vi "Sequence Dialog.vi"(8 "error in (no error)":errorcluster, 10 "Sequence UI":refnum<queue>, 11 "State Cluster In":T3 {"Main Config"."PR Module Configs"."Settings"."PID 2 Parameters"."output range"."output low" format="%.2f"; "Main Config"."PR Module Configs"."Settings"."PID 2 Parameters"."output range"."output high" min=0.0 max=100.0 format="%.2f"; "Main Config"."PR Module Configs"."Settings"."PID 2 Parameters"."PID gains"."derivative time (Td, min)" format="%.3f"; "Main Config"."PR Module Configs"."Settings"."PID 2 Parameters"."PID gains"."integral time (Ti, min)" format="%.3f"; "Main Config"."PR Module Configs"."Settings"."PID 2 Parameters"."PID gains"."proportional gain (Kc)" format="%.3f"; "Main Config"."Steps"."Control" items=["Pump %", "Setpoint"]; "Main Config"."TCU Module Configs"."Settings"."Huber Unistat 410 Settings"."Address" min=0 max=99 format="%02.0f"; "Main Config"."TCU Module Configs"."Settings"."Julabo FP-50 Settings"."Pump Power" min=0 max=8 step=1; "Main Config"."TCU Module Configs"."Settings"."Lauda Settings"."Pump Power" min=0 max=8 step=1; "Main Config"."Flow Module Configs"."Settings"."Bronkhorst M14 Settings"."Smoothing Steps" min=1 step=1; "Main Config"."Flow Module Configs"."Settings"."Bronkhorst M13 Settings"."Smoothing Steps" min=1 step=1; "Main Config"."Pump Module Configs"."Settings"."Ismatech 3 Channel Settings"."Channel Number" min=0 max=3; "Main Config"."Pump Module Configs"."Settings"."Ismatech 3 Channel Settings"."Pump Number" min=1; "Main Config"."Pump Module Configs"."Settings"."ASIA Pump C"."channel" min=0 max=1 step=1; "Main Config"."Pump Module Configs"."Settings"."Masterflex"."Pump Number" min=1.0 max=20.0 step=1.0; "Main Config"."Pump Module Configs"."Settings"."Ismatech"."Pump Number" min=1.0 max=20.0 step=1.0; "Main Config"."Feed Module Configs"."Settings"."Bronkhorst M14 Settings"."Smoothing Steps" min=1 step=1; "Main Config"."Feed Module Configs"."Settings"."Ismatech 3 Channel Settings"."Channel Number" min=0 max=3; "Main Config"."Feed Module Configs"."Settings"."Ismatech 3 Channel Settings"."Pump Number" min=1; "Main Config"."Feed Module Configs"."Settings"."PID range"."PID Low" min=0.0 max=100.0 format="%.2f"; "Main Config"."Feed Module Configs"."Settings"."PID range"."PID High" format="%.2f"; "Main Config"."Feed Module Configs"."Settings"."PID 2 Parameters"."PID gains"."derivative time (Td, min)" format="%.3f"; "Main Config"."Feed Module Configs"."Settings"."PID 2 Parameters"."PID gains"."integral time (Ti, min)" format="%.3f"; "Main Config"."Feed Module Configs"."Settings"."PID 2 Parameters"."PID gains"."proportional gain (Kc)" format="%.3f"; "Main Config"."Feed Module Configs"."Settings"."Bronkhorst M13 Flow Meter"."Smoothing Steps" min=1 step=1; "Main Config"."Feed Module Configs"."Settings"."ASIA Pump C"."channel" min=0 max=1 step=1; "Main Config"."Feed Module Configs"."Settings"."Ismatech"."Pump Number" min=1.0 max=20.0 step=1.0; "Main Config"."Feed Module Configs"."Settings"."Masterflex"."Pump Number" min=1.0 max=20.0 step=1.0}) -> (0 "error out":errorcluster, 1 "Start":bool, 2 "cancelled":bool, 3 "State Cluster Out":T3 {"Main Config"."PR Module Configs"."Settings"."PID 2 Parameters"."output range"."output low" format="%.2f"; "Main Config"."PR Module Configs"."Settings"."PID 2 Parameters"."output range"."output high" min=0.0 max=100.0 format="%.2f"; "Main Config"."PR Module Configs"."Settings"."PID 2 Parameters"."PID gains"."derivative time (Td, min)" format="%.3f"; "Main Config"."PR Module Configs"."Settings"."PID 2 Parameters"."PID gains"."integral time (Ti, min)" format="%.3f"; "Main Config"."PR Module Configs"."Settings"."PID 2 Parameters"."PID gains"."proportional gain (Kc)" format="%.3f"; "Main Config"."Steps"."Control" items=["Pump %", "Setpoint"]; "Main Config"."TCU Module Configs"."Settings"."Huber Unistat 410 Settings"."Address" min=0 max=99 format="%02.0f"; "Main Config"."TCU Module Configs"."Settings"."Julabo FP-50 Settings"."Pump Power" min=0 max=8 step=1; "Main Config"."TCU Module Configs"."Settings"."Lauda Settings"."Pump Power" min=0 max=8 step=1; "Main Config"."Flow Module Configs"."Settings"."Bronkhorst M14 Settings"."Smoothing Steps" min=1 step=1; "Main Config"."Flow Module Configs"."Settings"."Bronkhorst M13 Settings"."Smoothing Steps" min=1 step=1; "Main Config"."Pump Module Configs"."Settings"."Ismatech 3 Channel Settings"."Channel Number" min=0 max=3; "Main Config"."Pump Module Configs"."Settings"."Ismatech 3 Channel Settings"."Pump Number" min=1; "Main Config"."Pump Module Configs"."Settings"."ASIA Pump C"."channel" min=0 max=1 step=1; "Main Config"."Pump Module Configs"."Settings"."Masterflex"."Pump Number" min=1.0 max=20.0 step=1.0; "Main Config"."Pump Module Configs"."Settings"."Ismatech"."Pump Number" min=1.0 max=20.0 step=1.0; "Main Config"."Feed Module Configs"."Settings"."Bronkhorst M14 Settings"."Smoothing Steps" min=1 step=1; "Main Config"."Feed Module Configs"."Settings"."Ismatech 3 Channel Settings"."Channel Number" min=0 max=3; "Main Config"."Feed Module Configs"."Settings"."Ismatech 3 Channel Settings"."Pump Number" min=1; "Main Config"."Feed Module Configs"."Settings"."PID range"."PID Low" min=0.0 max=100.0 format="%.2f"; "Main Config"."Feed Module Configs"."Settings"."PID range"."PID High" format="%.2f"; "Main Config"."Feed Module Configs"."Settings"."PID 2 Parameters"."PID gains"."derivative time (Td, min)" format="%.3f"; "Main Config"."Feed Module Configs"."Settings"."PID 2 Parameters"."PID gains"."integral time (Ti, min)" format="%.3f"; "Main Config"."Feed Module Configs"."Settings"."PID 2 Parameters"."PID gains"."proportional gain (Kc)" format="%.3f"; "Main Config"."Feed Module Configs"."Settings"."Bronkhorst M13 Flow Meter"."Smoothing Steps" min=1 step=1; "Main Config"."Feed Module Configs"."Settings"."ASIA Pump C"."channel" min=0 max=1 step=1; "Main Config"."Feed Module Configs"."Settings"."Ismatech"."Pump Number" min=1.0 max=20.0 step=1.0; "Main Config"."Feed Module Configs"."Settings"."Masterflex"."Pump Number" min=1.0 max=20.0 step=1.0}, 4 "Pause":bool, 5 "Abort":bool)   [LabVIEW 2018, in "Sequencing Library.lvlib"]
uses:
  Sequencing Library.lvlib
  Squence Control.ctl
  controls/Step Cluster.ctl
  Drag and Drop/State Cluster.ctl
  support/Message Queue/Message Cluster.ctl
  Drag and Drop/Thumbnail Cluster.ctl
  Drag and Drop/Object Cluster.ctl
  <vilib>/Utility/miscctls.llb/LVRectTypeDef.ctl
  Drag and Drop/Object Type Enum.ctl
  <vilib>/Utility/miscctls.llb/LVPositionTypeDef.ctl
  Config Module/Controls/Main Config Cluster.ctl
  OPC/OPC Module Config.ctl
  Scale Module Folder/Measure Instrument/State Enum.ctl
  <vilib>/Utility/miscctls.llb/LVPoint32TypeDef.ctl
  OPC/OPC Settings.ctl
  OPC/Variable Data Cluster.ctl
  <vilib>/OPCUA/controls/NodeId.ctl
  <vilib>/OPCUA/controls/OPC UA StatusCode.ctl
  <vilib>/OPCUA/controls/Subscription ID.ctl
  <vilib>/OPCUA/controls/OPC UA Client Refnum.ctl
  <vilib>/OPCUA/controls/Subscription Data Change.ctl
  <vilib>/OPCUA/controls/Data Type.ctl
  OPC/OPC Tag Data.ctl
  Feed Module/Controls/Feed Module Config Cluster.ctl
  Feed Module/Controls/Feed Module Settings Cluster.ctl
  Ismatec ISM 831C/Controls/Ismatech ISM831C Settings Cluster.ctl
  Masterflex 7550-30/Controls/Settings Cluster.ctl
  Mettler Toledo/Controls/Settings Cluster.ctl
  Bronkhorst M13 Flow Meter/Settings Cluster.ctl
  Measure Instrument/PID 2 Parameters Cluster.ctl
  Measure Instrument/PID Input Enum.ctl
  Measure Instrument/PID 2 Output Enum.ctl
  Tacmina QI/Tacmina QI DAQ Setting.ctl
  KNF Pump/Settings Cluster plus SIMDOS.ctl
  ASIA Pump/Pump Settings.ctl
  VICI M50 Party Mode/Settings Cluster.ctl
  FLOM Pump/Settings Cluster.ctl
  SSI PR Class/SSI PR or LD Settings Cluster.ctl
  Masterflex 75211/Masterflex 75211 DAQ Setting.ctl
  SSI PR Class/SSI P40 Settings Cluster.ctl
  Ismatec 78001/Ismatec 4083.ctl
  Bronkhorst M14 Flow Meter/Settings Cluster.ctl
  Tag VIs/Numeric Alarm Settings Cluster.ctl
  TT Module/Controls/TT Module Config Cluster.ctl
  Acquisition/Hardware Configuration.ctl
  Acquisition/Task Cluster.ctl
  PT Module/Controls/PT Module Config Cluster.ctl
  Scale Module Folder/Feed Module/Controls/Scale Module Config Cluster.ctl
  Scale Module Folder/Feed Module/Controls/Scale Module Settings Cluster.ctl
  Pump Module Folder/Pump Module Config Cluster.ctl
  Pump Module Folder/Pump Module Settings Cluster.ctl
  LabJack Module/Controls/U3 Module Config Cluster.ctl
  Decoration Module/Decoration Module Config Cluster.ctl
  Flow Module Folder/Feed Module/Controls/Flow Module Config Cluster.ctl
  Flow Module Folder/Feed Module/Controls/Flow Module Settings Cluster.ctl
  TCU Module/TCU Module Folder/TCU Module Config Cluster.ctl
  TCU Module/TCU Module Folder/TCU Module Settings Cluster.ctl
  TCU Module/TCU Module Folder/Measure Instrument/Output Devices.ctl
  Huber TCU/Huber Settings.ctl
  Lauda Integral XT-150 TCU/Lauda Settings.ctl
  Julabo Type 1 TCU/Julabo Type 1 TCU Folder/Julabo FP-50 Settings.ctl
  Huber Unistat 410 TCU/Huber Unistat 410 RS485 Settings.ctl
  D-O Module Folder/Not Sure Where this is Used.ctl
  D-O Module Folder/D-O Module Config Cluster.ctl
  D-O Module Folder/Valve Clusters.ctl
  D-O Module Folder/D-O Module Settings Cluster.ctl
  D-O Module Folder/D-O Device Settings Cluster.ctl
  VICI Electronic Actuator/VICI Electronic Actuator Settings.ctl
  Pressure Regulator Control Module/Pressure Regulator/Controls/4-20mA Module Config Cluster.ctl
  Pressure Regulator Control Module/Pressure Regulator/Controls/4-20mA Module Settings Cluster.ctl
  Pressure Transmitter/Pressure Transmitter Device Settings.ctl
  Pressure Reg Module/Pressure Regulator Device Settings.ctl
  Sonicator Module Folder/Feed Module/Controls/Sonicator Module Config Cluster.ctl
  Sonicator Module Folder/Feed Module/Controls/Sonicator Module Settings Cluster.ctl
  Sonic Systems P100/Sonic Systems P100 Settings.ctl
  Agitator Module Folder/Feed Module/Controls/Agitator Module Config Cluster.ctl
  Agitator Module Folder/Feed Module/Controls/Agitator Module Settings Cluster.ctl
  IKA EUROSTAR/IKA EUROSTAR Settings.ctl
  Centrifuge Module Folder/Centrifuge Module Config Cluster.ctl
  Centrifuge Module Folder/Centrifuge Module Settings Cluster.ctl
  EPOS4/Controls/Device Selection.ctl
  EPOS4/Controls/EPOS Communication Settings.ctl
  support/Message Queue/Enqueue Message (Single).vi
  support/Message Queue/Message Queue.lvlib
  Report Generation/Report Generation.lvlib
  Drag and Drop/Drag and Drop.lvlib
  Config Module/Config Module.lvlib
  TT Module/TT Module.lvlib
  Feed Module/Feed Module.lvlib
  Ismatec ISM 831C/Ismatec ISM 831C.lvlib
  Masterflex 7550-30/Masterflex 7550-30.lvlib
  Mettler Toledo/Mettler Toledo.lvlib
  Bronkhorst M13 Flow Meter/Bronkhorst M13 Flow Meter.lvlib
  Tacmina QI/Tacmina QI.lvlib
  KNF Pump/KNF SIMDOS.lvlib
  ASIA Pump.lvlib
  DAQ/DAQ.lvlib
  PT Module/PT Module.lvlib
  Scale Module Folder/Scale Module.lvlib
  Pump Module Folder/Pump Module.lvlib
  LabJack Module/U3 Module.lvlib
  Flow Module Folder/Flow Module.lvlib
  TCU Module/TCU Module Folder/TCU Module.lvlib
  Huber TCU/Huber Ministat 230 TCU.lvlib
  Lauda Integral XT-150 TCU/Lauda TCU.lvlib
  Julabo Type 1 TCU/Julabo Type 1 TCU Folder/Julabo Type FP-50 TCU.lvlib
  VICI M50 Party Mode/VICI M6 M50 Party Mode.lvlib
  D-O Module Folder/D-O Module.lvlib
  Pressure Transmitter/Pressure Transmitter Library.lvlib
  Pressure Regulator Control Module/Pressure Regulator/4-20mA Module.lvlib
  Pressure Reg Module/Pressure Regulator Library.lvlib
  FLOM Pump/FLOM Pump.lvlib
  SSI PR Class/SSI PR or LD Pump.lvlib
  OPC/OPC UA.lvlib
  Scale Module Folder/Measure Instrument/Scale Module Engine.lvlib
  D-O Module Folder/DIO Valve/VICI Electronic Actuator.lvlib
  Masterflex 75211/Masterflex 75211.lvlib
  SSI PR Class/SSI P40 Pump.lvlib
  Huber Unistat 410 TCU/Huber Unistat 410 TCU.lvlib
  Ismatec 78001/Ismatec 4308.lvlib
  Bronkhorst M14 Flow Meter/Bronkhorst M14 Flow Meter.lvlib
  Sonicator Module Folder/Sonicator Module.lvlib
  Sonic Systems P100/Sonic Systems P100.lvlib
  Agitator Module Folder/Agitator Module.lvlib
  EPOS4/EPOS4.lvlib
  Centrifuge Module Folder/Centrifuge Module.lvlib
  IKA EUROSTAR/IKA EUROSTAR.lvlib
panel:
  out "Main Config.Steps":T1 {"Control" items=["Pump %", "Setpoint"]}
  out "Strings []":string[](array[string])
  in  "Abort  Button":bool
  in  "Pause Button":bool
  in  "Save Button":bool
  in  "Step Array":T78[](array[typedef]) {"Value" min=0.0 max=100.0; "Control" items=["Pump Module Setpoint", "Feed Module Setpoint", "Sonicator Module Setpoint", "Digital On/Off", "Wait Until Output <=", "Wait Until Output >=", "TCU Pump Setpoint", "TCU Temperature Setpoint", "Wait until TCU Temp <=", "Wait until TCU Temp >=", "Agitator Setpoint", "Centrifuge Setpoint", "Totalized Value", "Default"]; "Module" items=["Default", "Loop Start", "Loop End"]}
  out "Steps out":T2[](array[typedef]) {"Control" items=["Setpoint", "Pump %"]}
  in  "Cancel Button":bool
  in  "Start Button":bool
  # "Module"
  # "Control"
  # "Value"
  # "Wait (sec)"
  # "Running"
  # "Agitator Settings"
  # "Sonicator Settings"
  # "Instrument Settings"
  # "Instrument Settings"
  # "Output Instruments"
  # "Flow Meter Settings"
  # "Output Instruments"
  # "Scale Settings"
  # "Output Instruments"
  # "Input Instruments"
  # "Agitator Settings"
  # "Sonicator Settings"
  # "Instrument Settings"
  # "Instrument Settings"
  # "Output Instruments"
  # "Flow Meter Settings"
  # "Output Instruments"
  # "Scale Settings"
  # "Output Instruments"
  # "Input Instruments"
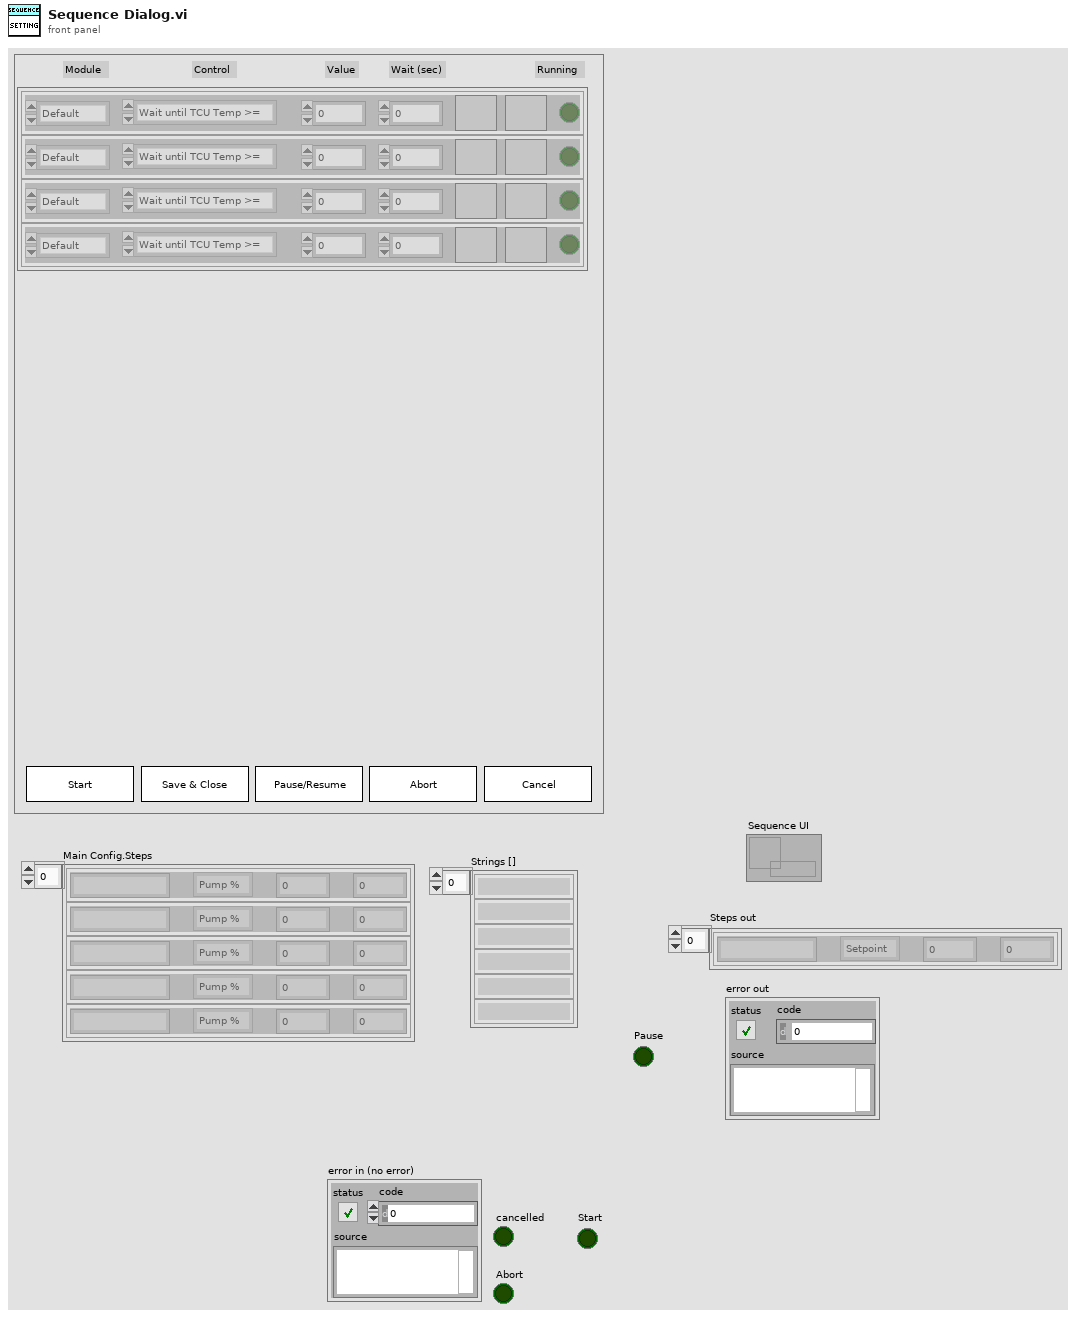
[diagram p1: front panel]
types:
  T1 = typedef "Not Sure Where this is Used.ctl" = T2[]
  T2 = typedef "Sequencing Library.lvlib/Squence Control.ctl" = cluster{"Module":string, "Control":u16, "Value":dbl, "Wait (sec)":dbl}
  T3 = typedef "Drag and Drop.lvlib/State Cluster.ctl" = cluster{"VI refs":refnum<vi>[], "Queues":refnum<queue>[], "[Thumbnails]":T4[], "Drag Object Idx":i32, "[Objects]":T5[], "Active Object":i32, "Drop Offset":T8, "Process Name":string, "Main Config":T9, "Campaign Filepath":path, "Config Changed?":bool}
  T4 = typedef "Thumbnail Cluster.ctl" = cluster{"Path":path, "Rectangle":cluster{"left":i16, "top":i16, "right":i16, "bottom":i16}}
  T5 = typedef "Object Cluster.ctl" = cluster{"BMP Path":path, "Anchor Position":cluster{"X":i32, "Y":i32}, "Hot Spot":T6, "Type":T7, "Parameters":variant}
  T6 = typedef "LVRectTypeDef.ctl" = cluster{"Left":i16, "Top":i16, "Right":i16, "Bottom":i16}
  T7 = typedef "Object Type Enum.ctl" = enum16{"Icon", "Line", "Text", "Feed Module"}
  T8 = typedef "LVPositionTypeDef.ctl" = cluster{"Left":i32, "Top":i32}
  T9 = typedef "Config Module.lvlib/Main Config Cluster.ctl" = cluster{"Notebook":string, "OPC Module Configs":T10[], "Feed Module Configs":T20[], "Log File Path":path, "TT Module Configs":T40[], "DAQ Config":T41, "PT Module Configs":T43[], "Scale Module Configs":T44[], "Pump Module Configs":T46[], "U3 Module Configs":T48[], "Decoration Module Configs":T49[], "Flow Module Configs":T50[], "TCU Module Configs":T52[], "Steps":T1, "Abort":bool, "DO Module Configs":T59[], "PR Module Configs":T64[], "SC Module Configs":T68[], "AM Module Configs":T71[], "CM Module Configs":T74[], "Cycle Period":dbl}
  T10 = typedef "OPC UA.lvlib/OPC Module Config.ctl" = cluster{"State":T11, "GUID":string, "Process Name":string, "User name":string, "Drop Coords":T12, "Configuration":T13, "First Iteration":bool, "Data":cluster{"Object Name":string, "Variable Array":T14[]}[], "Load Count":i32, "Log Started":bool, "subscription ID out":T17, "OPC UA client refnum out":T18, "Event Registration Refnum":refnum<event-registration>, "Start Time":timestamp, "Current Time":timestamp, "Tag Data":T19[]}
  T11 = typedef "Scale Module.lvlib/Scale Module Engine.lvlib/State Enum.ctl" = enum16{"Measuring", "Idle"}
  T12 = typedef "LVPoint32TypeDef.ctl" = cluster{"Horizontal":i32, "Vertical":i32}
  T13 = typedef "OPC UA.lvlib/OPC Settings.ctl" = cluster{"Cycle Period":dbl, "server endpoint URL":string, "security policy":cluster{"message mode":enum16{"None", "Sign", "Sign and Encrypt"}, "security":enum16{"Basic256", "Basic128Rsa15"}}, "Trust Any Server":bool}
  T14 = typedef "OPC UA.lvlib/Variable Data Cluster.ctl" = cluster{"node ID":T15, "browse name":string, "status":T16, "timestamp":timestamp, "value ":variant}
  T15 = typedef "NodeId.ctl" = string
  T16 = typedef "OPC UA StatusCode.ctl" = u32
  T17 = typedef "Subscription ID.ctl" = u32
  T18 = typedef "OPC UA Client Refnum.ctl" = refnum<k21>
  T19 = typedef "OPC UA.lvlib/OPC Tag Data.ctl" = cluster{"Include this Device":bool, "Device Name":string, "OPC Tag Data":cluster{"Tag":string, "Value":variant, "Time Stamp":timestamp}[]}
  T20 = typedef "Feed Module.lvlib/Feed Module Config Cluster.ctl" = cluster{"GUID":string, "Drop Coords":T12, "Process Name":string, "User name":string, "Queue Name":string, "Settings":T21, "Settings Load Count":i32, "OP Load Count":i32}
  T21 = typedef "Feed Module.lvlib/Feed Module Settings Cluster.ctl" = cluster{"Cycle Period":dbl, "Ismatech":T22, "Masterflex":T23, "Mettler":T24, "Bronkhorst M13 Flow Meter":T25, "PID 2 Parameters":T26, "Manual Entry":dbl, "Auto?":bool, "PID range":cluster{"PID High":dbl, "PID Low":dbl, "High Warning":dbl}, "Tacmina Settings":T29, "KNF SIMDOS Settings":T30, "ASIA Pump C":T31, "VICI Settings":T32, "FLOM Settings":T33, "SSI PR/LD Settings":T34, "Masterflex 75211 Settings":T35, "SSI P40 Settings":T36, "Ismatech 3 Channel Settings":T37, "Bronkhorst M14 Settings":T38, "Reset Totalizer":bool, "Input Num Alarm Settings":T39[], "Control Type":enum32{"g/min", "ml/min"}, "Front End Display Options":cluster{"Temperature":bool, "Scale Grams":bool, "Density":bool, "Flow (g/min)":bool, "Flow (ml/min)":bool, "PSIG":bool, "Total Grams":bool, "Updated":bool}}
  T22 = typedef "Ismatec ISM 831C.lvlib/Ismatech ISM831C Settings Cluster.ctl" = cluster{"VISA resource name":refnum<visa-resource-name>, "Simulated?":bool, "Pump Number":dbl, "Reverse?":bool}
  T23 = typedef "Masterflex 7550-30.lvlib/Settings Cluster.ctl" = cluster{"VISA resource name":refnum<visa-resource-name>, "Simulated?":bool, "Pump Number":dbl, "Reverse?":bool}
  T24 = typedef "Mettler Toledo.lvlib/Settings Cluster.ctl" = cluster{"VISA resource name":refnum<visa-resource-name>, "Simulated?":bool}
  T25 = typedef "Bronkhorst M13 Flow Meter.lvlib/Settings Cluster.ctl" = cluster{"VISA resource name":refnum<visa-resource-name>, "Simulated?":bool, "Smoothing Steps":i32}
  T26 = typedef "PID 2 Parameters Cluster.ctl" = cluster{"Input Device":T27, "Output Device":T28, "Setpoint":dbl, "PID gains":cluster{"proportional gain (Kc)":dbl, "integral time (Ti, min)":dbl, "derivative time (Td, min)":dbl}}
  T27 = typedef "PID Input Enum.ctl" = enum16{"Default", "Bronkhorst M13", "Bronkhorst M14", "Scale Rate of Change"}
  T28 = typedef "PID 2 Output Enum.ctl" = enum16{"Default", "Ismatec ISM 4308", "Ismatec ISM 831C", "Masterflex 7550-30", "VICI M6", "VICI M50", "Tacmina QI", "KNF SIMDOS", "ASIA Type C", "FLOM UI-22-11", "SSI PR/LD", "SSI P40", "Masterflex 75211-70"}
  T29 = typedef "Tacmina QI.lvlib/Tacmina QI DAQ Setting.ctl" = cluster{"Analog DAQ Task":refnum<k21>, "Digital DAQ Task":refnum<k21>}
  T30 = typedef "KNF SIMDOS.lvlib/Settings Cluster plus SIMDOS.ctl" = cluster{"VISA resource name":refnum<visa-resource-name>, "Simulated?":bool}
  T31 = typedef "ASIA Pump.lvlib/Pump Settings.ctl" = cluster{"ASIA Pump #":i32, "channel":i32, "Simulated":bool}
  T32 = typedef "VICI M6 M50 Party Mode.lvlib/Settings Cluster.ctl" = cluster{"VISA resource name":refnum<visa-resource-name>, "Pump ID":string, "Pump Head Vol":dbl, "Reverse?":bool, "Simulated?":bool}
  T33 = typedef "FLOM Pump.lvlib/Settings Cluster.ctl" = cluster{"VISA resource name":refnum<visa-resource-name>, "Simulated?":bool, "Pump Number":dbl}
  T34 = typedef "SSI PR or LD Pump.lvlib/SSI PR or LD Settings Cluster.ctl" = cluster{"VISA resource name":refnum<visa-resource-name>, "Simulated?":bool}
  T35 = typedef "Masterflex 75211.lvlib/Masterflex 75211 DAQ Setting.ctl" = cluster{"Analog DAQ Task":refnum<k21>, "Digital DAQ Task":refnum<k21>}
  T36 = typedef "SSI P40 Pump.lvlib/SSI P40 Settings Cluster.ctl" = cluster{"VISA resource name":refnum<visa-resource-name>, "Simulated?":bool}
  T37 = typedef "Ismatec 4308.lvlib/Ismatec 4083.ctl" = cluster{"VISA resource name":refnum<visa-resource-name>, "Pump Number":i16, "Channel Number":i16, "Simulated?":bool, "Reverse?":bool}
  T38 = typedef "Bronkhorst M14 Flow Meter.lvlib/Settings Cluster.ctl" = cluster{"VISA resource name":refnum<visa-resource-name>, "Simulated?":bool, "Smoothing Steps":i32}
  T39 = typedef "Numeric Alarm Settings Cluster.ctl" = cluster{"enable? (F)":bool, "name":string, "alarm type":enum16{"HI_HI", "HI", "LO", "LO_LO"}, "level/change":dbl, "deadband/time":dbl, "alarm delay":dbl, "priority":u32, "ack type":enum16{"Auto", "User", "None", "Each Occurrence"}, "area":string, "description":string, "log? (T)":bool}
  T40 = typedef "TT Module.lvlib/TT Module Config Cluster.ctl" = cluster{"GUID":string, "Drop Coords":T12, "Input Channel Tag Name ":string, "Process Name":string, "User name":string, "Queue Name":string, "Input Channel Numeric Alarm Settings":T39[]}
  T41 = typedef "DAQ.lvlib/Hardware Configuration.ctl" = cluster{"Tasks Array":T42[]}
  T42 = typedef "Task Cluster.ctl" = cluster{"DAQmx Task":refnum<k21>, "Read-Write Radio":enum32{"Read", "Write"}}
  T43 = typedef "PT Module.lvlib/PT Module Config Cluster.ctl" = cluster{"GUID":string, "Drop Coords":T12, "Input Channel Tag Name ":string, "Process Name":string, "User name":string, "Queue Name":string, "Input Channel Numeric Alarm Settings":T39[]}
  T44 = typedef "Scale Module.lvlib/Scale Module Config Cluster.ctl" = cluster{"GUID":string, "Drop Coords":T12, "Process Name":string, "User name":string, "Queue Name":string, "Settings":T45, "Load Count":i32}
  T45 = typedef "Scale Module.lvlib/Scale Module Settings Cluster.ctl" = cluster{"Cycle Period":dbl, "Mettler":T24, "Scale Type":string}
  T46 = typedef "Pump Module.lvlib/Pump Module Config Cluster.ctl" = cluster{"GUID":string, "Drop Coords":T12, "Process Name":string, "User name":string, "Queue Name":string, "Settings":T47, "Load Count":i32}
  T47 = typedef "Pump Module.lvlib/Pump Module Settings Cluster.ctl" = cluster{"Cycle Period":dbl, "Manual Entry":dbl, "Output Device":T28, "Ismatech":T22, "Ismatech 3 Channel Settings":T37, "Masterflex":T23, "VICI Settings":T32, "Tacmina Settings":T29, "KNF SIMDOS Settings":T30, "ASIA Pump C":T31, "FLOM Settings":T33, "SSI PR/LD Settings":T34, "SSI P40 Settings":T34, "Masterflex 75211 Settings":T35, "Pump Calibration File":path, "Calibration Slope":dbl, "Calibration Y Intercept":dbl, "Pump Cal Enum":u16, "Reset Totalizer":bool}
  T48 = typedef "U3 Module.lvlib/U3 Module Config Cluster.ctl" = cluster{"GUID":string, "Drop Coords":T12, "AI Channel Number":enum16{"Default", "AI0", "AI1", "AI2", "AI3", "AI4", "AI5", "AI6", "AI7"}, "Process Name":string, "User name":string, "Queue Name":string, "Input Channel Numeric Alarm Settings":T39[]}
  T49 = typedef "Decoration Module Config Cluster.ctl" = cluster{"GUID":string, "Drop Coords":T12, "Decoration Filepath":path}
  T50 = typedef "Flow Module.lvlib/Flow Module Config Cluster.ctl" = cluster{"GUID":string, "Drop Coords":T12, "Process Name":string, "User name":string, "Queue Name":string, "Settings":T51, "Load Count":i32}
  T51 = typedef "Flow Module.lvlib/Flow Module Settings Cluster.ctl" = cluster{"Cycle Period":dbl, "Flow Meter Type":string, "Bronkhorst M13 Settings":T25, "Bronkhorst M14 Settings":T38, "Reset Totalizer":bool}
  T52 = typedef "TCU Module.lvlib/TCU Module Config Cluster.ctl" = cluster{"GUID":string, "Drop Coords":T12, "Process Name":string, "User name":string, "Queue Name":string, "Settings":T53, "Load Count":i32, "Power Level Changed":bool}
  T53 = typedef "TCU Module.lvlib/TCU Module Settings Cluster.ctl" = cluster{"Cycle Period":dbl, "Setpoint Entry":dbl, "Output Device":T54, "Huber Ministat 230 Settings":T55, "Lauda Settings":T56, "Julabo FP-50 Settings":T57, "Internal Control?":bool, "Huber Unistat 410 Settings":T58}
  T54 = typedef "Output Devices.ctl" = enum16{"Default", "Huber Ministat 230", "Huber Unistat 410", "Lauda XT-150", "Julabo FP-50"}
  T55 = typedef "Huber Ministat 230 TCU.lvlib/Huber Settings.ctl" = cluster{"VISA resource name":refnum<visa-resource-name>, "Simulated?":bool}
  T56 = typedef "Lauda TCU.lvlib/Lauda Settings.ctl" = cluster{"VISA resource name":refnum<visa-resource-name>, "Simulated?":bool, "Pump Power":i32}
  T57 = typedef "Julabo Type FP-50 TCU.lvlib/Julabo FP-50 Settings.ctl" = cluster{"VISA resource name":refnum<visa-resource-name>, "Simulated?":bool, "Pump Power":i32}
  T58 = typedef "Huber Unistat 410 TCU.lvlib/Huber Unistat 410 RS485 Settings.ctl" = cluster{"VISA resource name":refnum<visa-resource-name>, "Address":i8, "Simulated?":bool}
  T59 = typedef "D-O Module.lvlib/D-O Module Config Cluster.ctl" = cluster{"GUID":string, "Drop Coords":T12, "Process Name":string, "User name":string, "Queue Name":string, "Settings":T60, "Load Count":i32}
  T60 = typedef "D-O Module.lvlib/Valve Clusters.ctl" = cluster{"Valve Settings":T61, "Valve Type":enum16{"Default", "Digital Output Valve", "VICI Electronic Actuator"}, "Time On (Sec)":dbl, "Time Off (Sec)":dbl, "Run?":bool}
  T61 = typedef "D-O Module.lvlib/D-O Module Settings Cluster.ctl" = cluster{"D-O Settings":T62, "VICI Electronic Actuator":T63}
  T62 = typedef "D-O Module.lvlib/D-O Device Settings Cluster.ctl" = cluster{"DAQmx Task Name":refnum<k21>, "Output Channel":u16, "Output Channel Names":string[]}
  T63 = typedef "VICI Electronic Actuator.lvlib/VICI Electronic Actuator Settings.ctl" = cluster{"VISA resource name":refnum<visa-resource-name>, "Mode":enum16{"Two Positions With Stops", "Two Positions Without Stops", "Mutiposition"}, "Simulated":bool}
  T64 = typedef "4-20mA Module.lvlib/4-20mA Module Config Cluster.ctl" = cluster{"GUID":string, "Drop Coords":T12, "Process Name":string, "User name":string, "Queue Name":string, "Settings":T65, "Settings Load Count":i32}
  T65 = typedef "4-20mA Module.lvlib/4-20mA Module Settings Cluster.ctl" = cluster{"Cycle Period":dbl, "PID 2 Parameters":cluster{"Input Device":enum16{"Default", "4-20mA"}, "Output Device":enum16{"Default", "Equilibar Pressure Reg", "Flow Regulator"}, "Setpoint":dbl, "PID gains":cluster{"proportional gain (Kc)":dbl, "integral time (Ti, min)":dbl, "derivative time (Td, min)":dbl}, "output range":cluster{"output low":dbl, "output high":dbl}}, "Manual Entry":dbl, "Auto?":bool, "4-20mA Input Settings":T66, "4-20mA Out Settings":T67, "Input Channel Tag Name ":string}
  T66 = typedef "Pressure Transmitter Library.lvlib/Pressure Transmitter Device Settings.ctl" = cluster{"Input Channel ":u16}
  T67 = typedef "Pressure Regulator Library.lvlib/Pressure Regulator Device Settings.ctl" = cluster{"Output DAQ Task":refnum<k21>}
  T68 = typedef "Sonicator Module.lvlib/Sonicator Module Config Cluster.ctl" = cluster{"GUID":string, "Drop Coords":T12, "Process Name":string, "User name":string, "Queue Name":string, "Settings":T69, "Load Count":i32}
  T69 = typedef "Sonicator Module.lvlib/Sonicator Module Settings Cluster.ctl" = cluster{"Cycle Period":dbl, "Sonicator Type":string, "SS P100 Settings":T70, "Setpoint (µm)":dbl, "Cutoff (W)":dbl}
  T70 = typedef "Sonic Systems P100.lvlib/Sonic Systems P100 Settings.ctl" = cluster{"VISA resource name":refnum<visa-resource-name>, "Simulated?":bool}
  T71 = typedef "Agitator Module.lvlib/Agitator Module Config Cluster.ctl" = cluster{"GUID":string, "Drop Coords":T12, "Process Name":string, "User name":string, "Queue Name":string, "Settings":T72, "Load Count":i32}
  T72 = typedef "Agitator Module.lvlib/Agitator Module Settings Cluster.ctl" = cluster{"Cycle Period":dbl, "Agitator Type":string, "Setpoint (µm)":dbl, "IKA EUROSTAR Settings":T73}
  T73 = typedef "IKA EUROSTAR.lvlib/IKA EUROSTAR Settings.ctl" = cluster{"VISA resource name":refnum<visa-resource-name>, "Simulated?":bool}
  T74 = typedef "Centrifuge Module.lvlib/Centrifuge Module Config Cluster.ctl" = cluster{"GUID":string, "Drop Coords":T12, "Process Name":string, "User name":string, "Queue Name":string, "Settings":T75, "Load Count":i32}
  T75 = typedef "Centrifuge Module.lvlib/Centrifuge Module Settings Cluster.ctl" = cluster{"Cycle Period":dbl, "Manual Entry":dbl, "Output Device":T76, "EPOS4 Settings":T77}
  T76 = typedef "Device Selection.ctl" = enum16{"Default", "EPOS4"}
  T77 = typedef "EPOS4.lvlib/EPOS Communication Settings.ctl" = cluster{"VISA resource name":refnum<visa-resource-name>, "axis":cluster{"keyHandle":u32, "nodeId":u16}, "Simulated?":bool}
  T78 = typedef "Sequencing Library.lvlib/Step Cluster.ctl" = cluster{"Add Button":bool, "Remove Button":bool, "Module":u16, "Control":u16, "Value":dbl, "Wait (sec)":dbl, "Step Running":bool}
  T79 = cluster{"Add Button":bool, "Remove Button":bool, "Module":u16, "Control":u16, "Value":dbl, "Wait (sec)":dbl, "Step Running":bool}
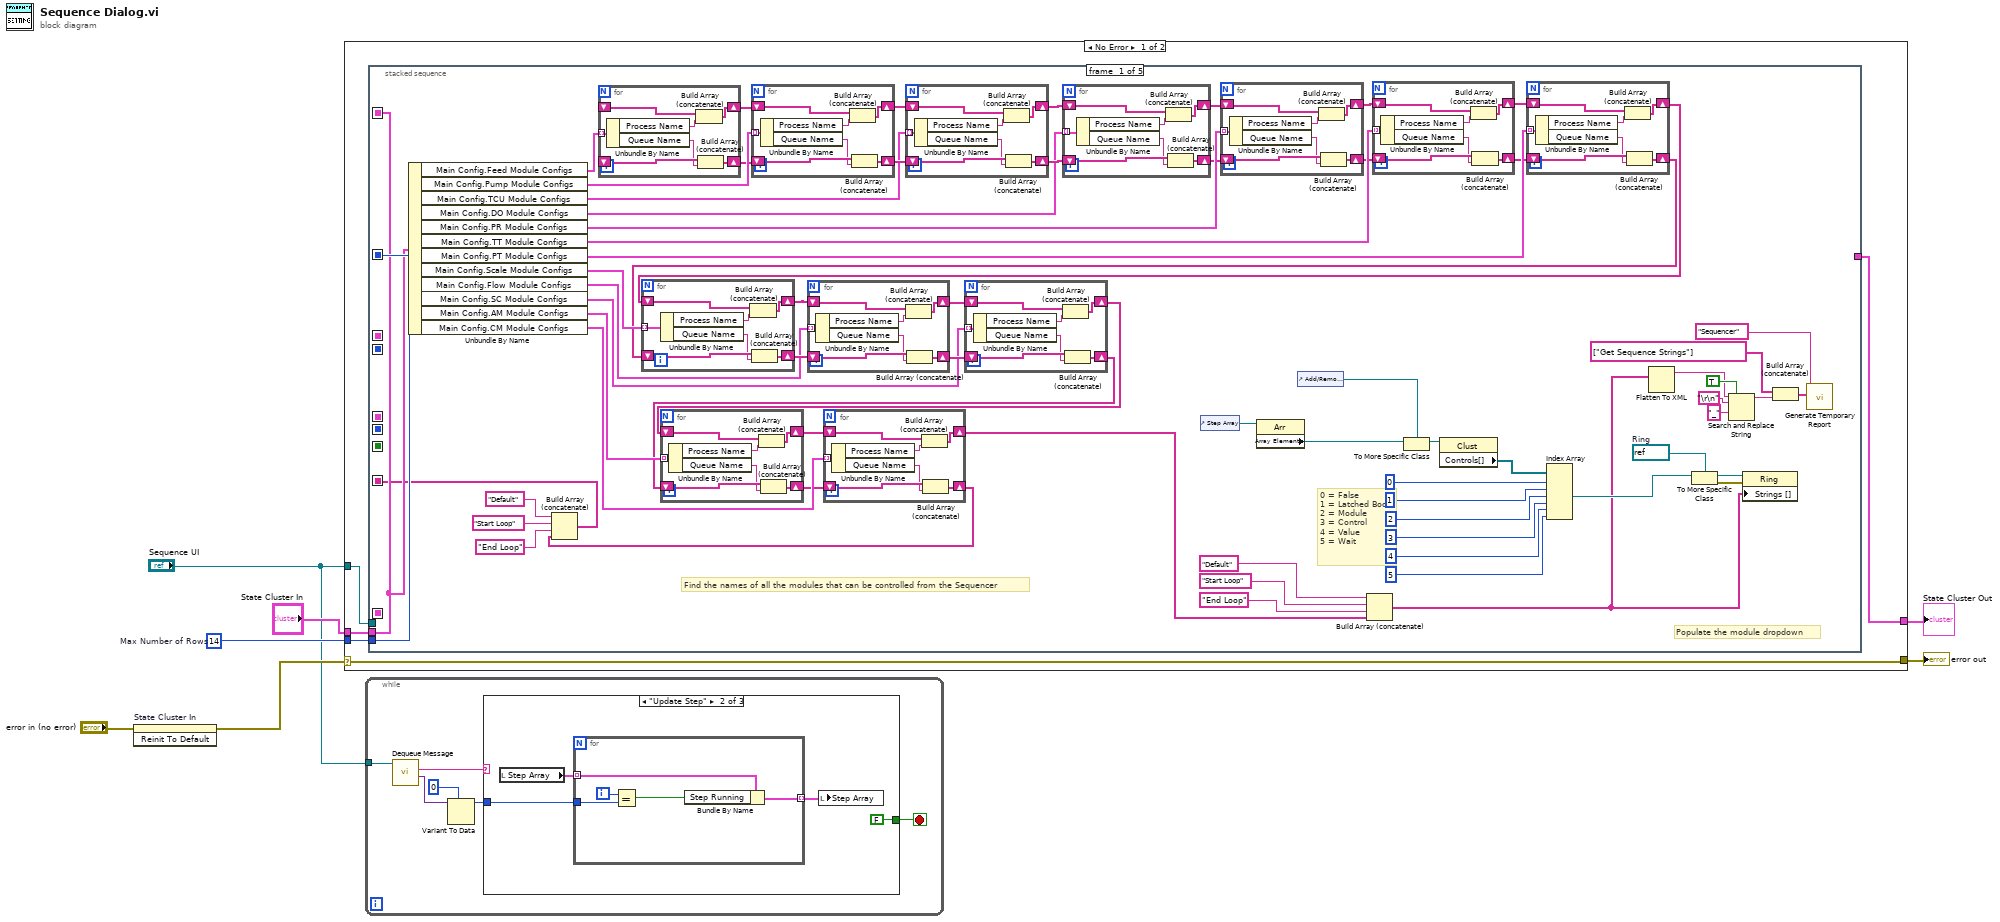
[diagram p0: block diagram]
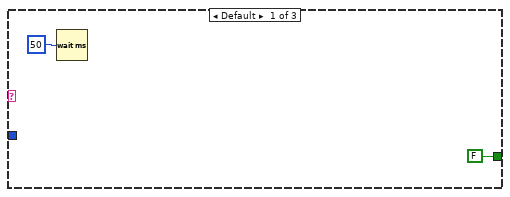
[diagram p2: hidden frame]
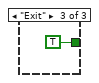
[diagram p3: hidden frame]
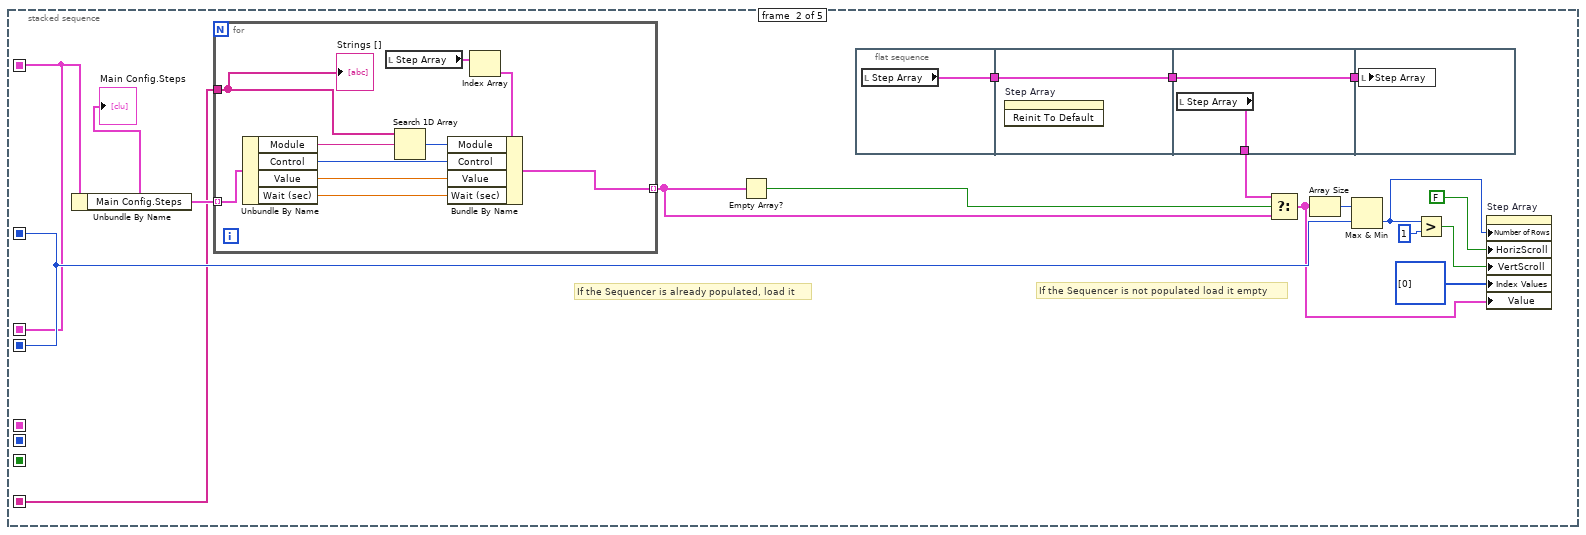
[diagram p4: hidden frame]
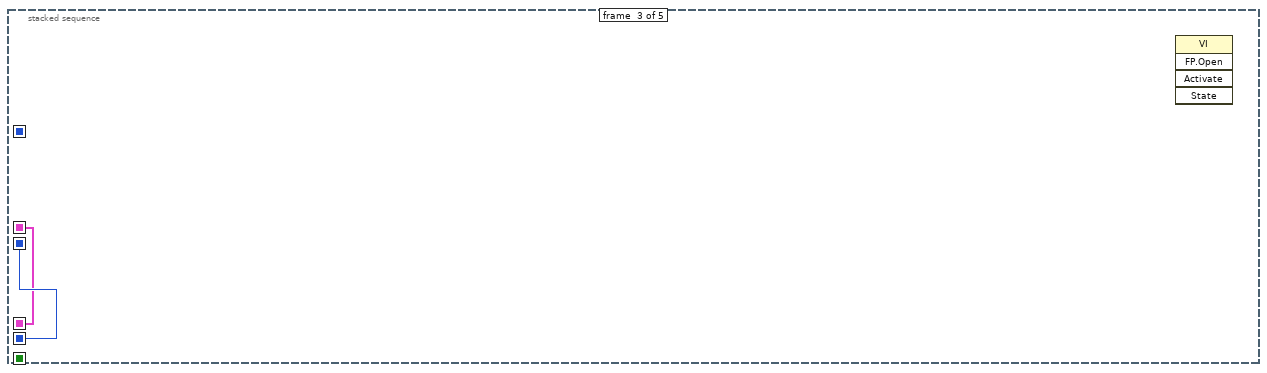
[diagram p5: hidden frame]
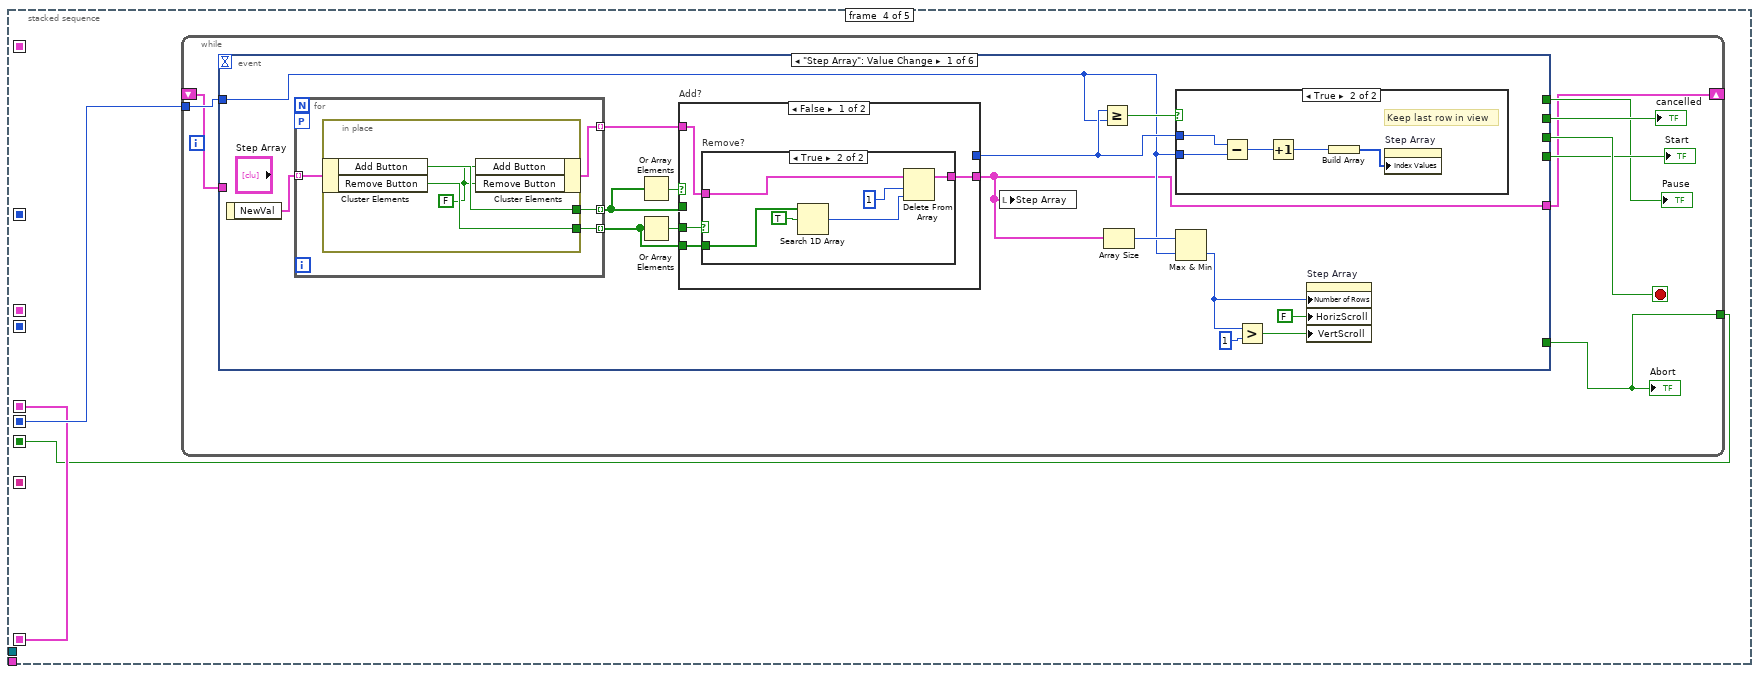
[diagram p6: hidden frame]
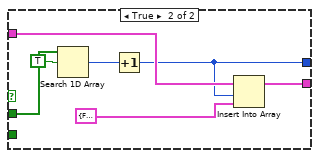
[diagram p9: hidden frame]
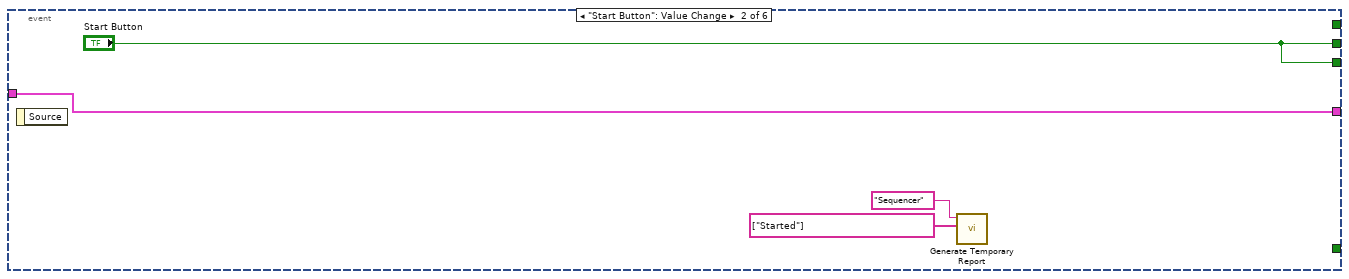
[diagram p10: hidden frame]
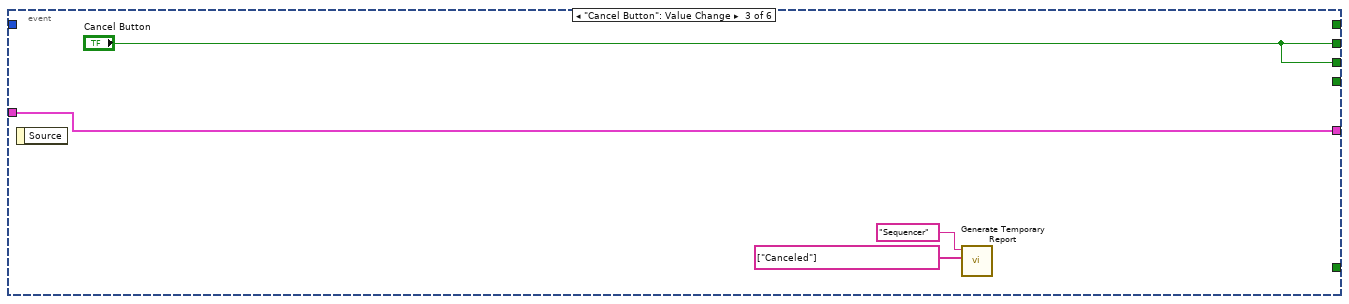
[diagram p11: hidden frame]
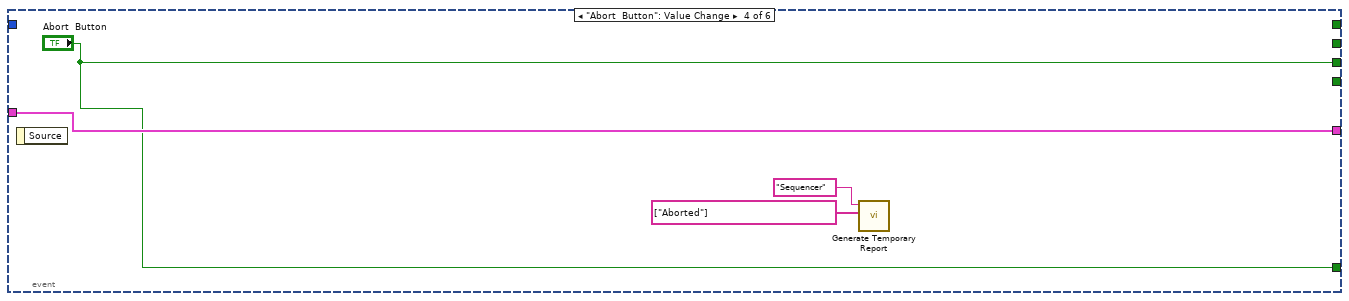
[diagram p12: hidden frame]
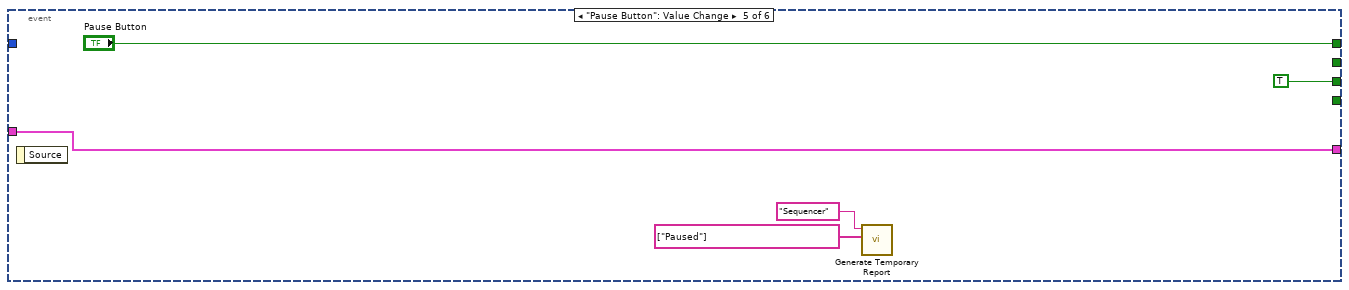
[diagram p13: hidden frame]
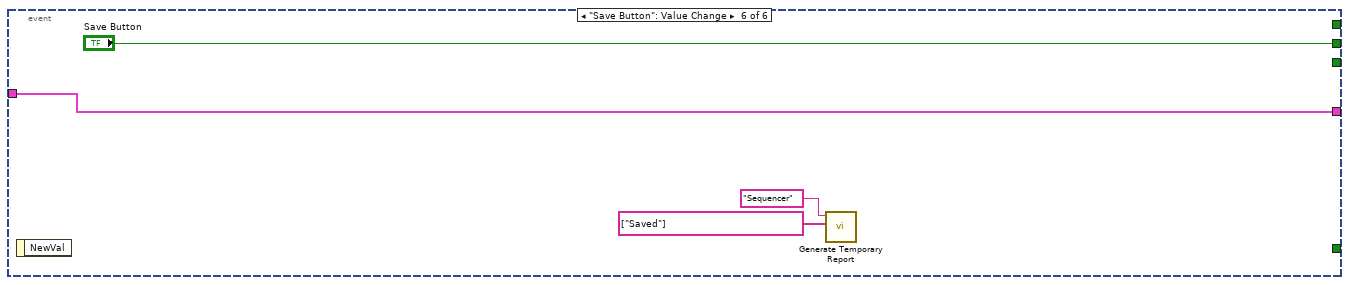
[diagram p14: hidden frame]
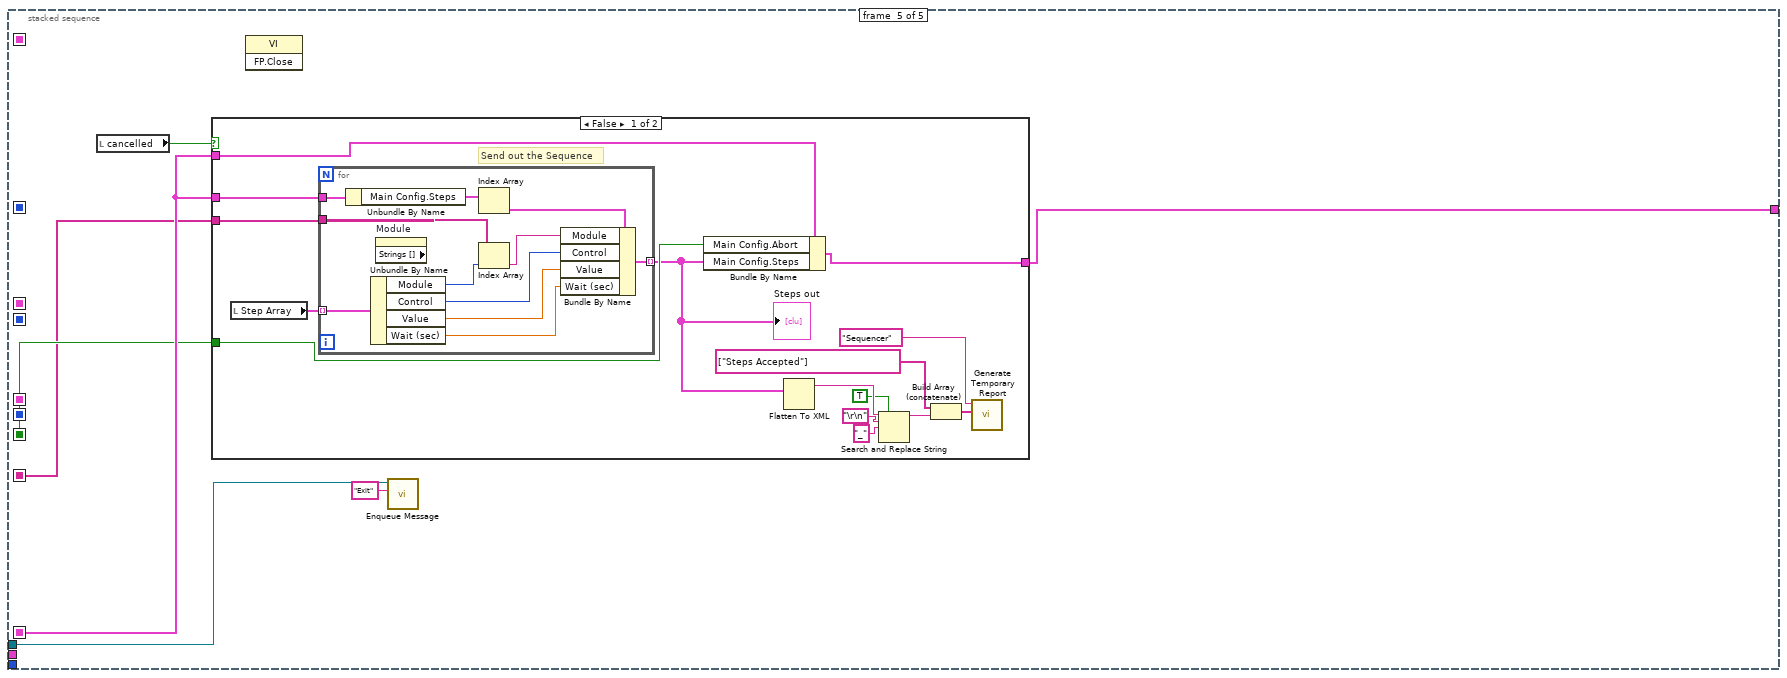
[diagram p15: hidden frame]
diagram:
  w6 = u32 14  # Max Number of Rows
  n1 = invoke on="State Cluster In" class="Clust (strict)" method="Reinit To Default"(error in="error in (no error)") -> (error out=w4:errorcluster)  [unwired: 2 in, 2 out]
  n2 = case shown="No Error" w4 {
    selector: w4 -> [w12 w312]
    tunnel: [w12 w312] -> w7
    tunnel: w6 -> [w11 _]
    tunnel: "State Cluster In" -> [w10 w311]
    tunnel: [w9 w311] -> w5
    tunnel: "Sequence UI" -> [w8 _]
    frame No Error {
      n3 = stacked-sequence {
        seq-local: [w80 _ _ _ _] -> [_ w179 _ _ _]
        seq-local: [w79 _ _ _ _] -> [_ w172 _ _ _]
        seq-local: [_ w179 _ _ _] -> [_ _ w199 _ _]
        seq-local: [_ w172 _ _ _] -> [_ _ w198 _ _]
        seq-local: [_ _ w199 _ _] -> [_ _ _ w202 _]
        seq-local: [_ _ w198 _ _] -> [_ _ _ w201 _]
        seq-local: [_ _ _ w201 _] -> [_ _ _ _ w281]
        seq-local: [_ _ _ w200 _] -> [_ _ _ _ w279]
        seq-local: [w35 _ _ _ _] -> [_ w166 _ _ w278]
        tunnel: w11 -> [w80 _ _ _ _]
        tunnel: w10 -> [w79 _ _ _ _]
        tunnel: [_ _ _ _ w282] -> w9
        tunnel: w8 -> [_ _ _ _ w277]
        frame #0 {
          w68 = refnum<vi> refnum  # Ring
          # "Populate the module dropdown"
          # "Find the names of all the modules that can be controlled from the Sequencer"
          # "0 = False\n1 = Latched Bool\n2 = Module\n3 = Control\n4 = Value\n5 = Wait"
          n4 = Unbundle By Name(w79) -> ("Main Config.Feed Module Configs"=w81:T20[], "Main Config.Pump Module Configs"=w60:T46[], "Main Config.TCU Module Configs"=w57:T52[], "Main Config.DO Module Configs"=w53:T59[], "Main Config.PR Module Configs"=w51:T64[], "Main Config.TT Module Configs"=w49:T40[], "Main Config.PT Module Configs"=w45:T43[], "Main Config.Scale Module Configs"=w40:T44[], "Main Config.Flow Module Configs"=w34:T50[], "Main Config.SC Module Configs"=w31:T68[], "Main Config.AM Module Configs"=w20:T71[], "Main Config.CM Module Configs"=w19:T74[])
          n5 = for {
            shift-right: [w162] -> w61
            shift-left: _ -> [w164]
            tunnel: w81 -> [w163] mode=indexing
            shift-right: [w161] -> w59
            shift-left: _ -> [w160]
            n6 = Unbundle By Name(w163) -> ("Process Name"=w165:string, "Queue Name"=w159:string)
            n7 = Build Array (concatenate)(w164, w165) -> (w162:string[])
            n8 = Build Array (concatenate)(w160, w159) -> (w161:string[])
          }
          n9 = for {
            shift-right: [w155] -> w56
            shift-left: w61 -> [w157]
            tunnel: w60 -> [w156] mode=indexing
            shift-right: [w154] -> w58
            shift-left: w59 -> [w153]
            n10 = Unbundle By Name(w156) -> ("Process Name"=w158:string, "Queue Name"=w152:string)
            n11 = Build Array (concatenate)(w157, w158) -> (w155:string[])
            n12 = Build Array (concatenate)(w153, w152) -> (w154:string[])
          }
          n13 = for {
            shift-right: [w148] -> w55
            shift-left: w56 -> [w150]
            tunnel: w57 -> [w149] mode=indexing
            shift-right: [w147] -> w54
            shift-left: w58 -> [w146]
            n14 = Unbundle By Name(w149) -> ("Process Name"=w151:string, "Queue Name"=w145:string)
            n15 = Build Array (concatenate)(w150, w151) -> (w148:string[])
            n16 = Build Array (concatenate)(w146, w145) -> (w147:string[])
          }
          n17 = for {
            shift-right: [w142] -> w52
            shift-left: w55 -> [w143]
            shift-right: [w141] -> w50
            shift-left: w54 -> [w140]
            tunnel: w53 -> [w138] mode=indexing
            n18 = Unbundle By Name(w138) -> ("Process Name"=w144:string, "Queue Name"=w139:string)
            n19 = Build Array (concatenate)(w143, w144) -> (w142:string[])
            n20 = Build Array (concatenate)(w140, w139) -> (w141:string[])
          }
          n21 = control-ref of="Step Array"() -> (w74:refnum<vi>)
          n22 = for {
            shift-right: [w134] -> w47
            shift-left: w52 -> [w136]
            tunnel: w51 -> [w135] mode=indexing
            shift-right: [w133] -> w48
            shift-left: w50 -> [w132]
            n23 = Unbundle By Name(w135) -> ("Process Name"=w137:string, "Queue Name"=w131:string)
            n24 = Build Array (concatenate)(w136, w137) -> (w134:string[])
            n25 = Build Array (concatenate)(w132, w131) -> (w133:string[])
          }
          n26 = property class="Arr"(reference=w74) -> ("Array Element"=w75:refnum<vi>)  [unwired: 1 in, 2 out]
          n27 = control-ref of="Add/Remove Cluster"() -> (w13:refnum<vi>)
          n28 = for {
            shift-right: [w127] -> w46
            shift-left: w47 -> [w129]
            tunnel: w49 -> [w128] mode=indexing
            shift-right: [w126] -> w44
            shift-left: w48 -> [w125]
            n29 = Unbundle By Name(w128) -> ("Process Name"=w130:string, "Queue Name"=w124:string)
            n30 = Build Array (concatenate)(w129, w130) -> (w127:string[])
            n31 = Build Array (concatenate)(w125, w124) -> (w126:string[])
          }
          n32 = To More Specific Class(target class=w13, reference=w75) -> (specific class reference=w76:refnum<vi>)  [unwired: 1 in, 1 out]
          n33 = property class="Clust"(reference=w76) -> ("Controls[]"=w69:refnum<vi>[])  [unwired: 1 in, 2 out]
          n34 = for {
            shift-right: [w120] -> w42
            shift-left: w46 -> [w122]
            tunnel: w45 -> [w121] mode=indexing
            shift-right: [w119] -> w39
            shift-left: w44 -> [w118]
            n35 = Unbundle By Name(w121) -> ("Process Name"=w123:string, "Queue Name"=w117:string)
            n36 = Build Array (concatenate)(w122, w123) -> (w120:string[])
            n37 = Build Array (concatenate)(w118, w117) -> (w119:string[])
          }
          n38 = for {
            shift-right: [w113] -> w43
            shift-left: w42 -> [w115]
            tunnel: w40 -> [w114] mode=indexing
            shift-right: [w112] -> w41
            shift-left: w39 -> [w111]
            n39 = Unbundle By Name(w114) -> ("Process Name"=w116:string, "Queue Name"=w110:string)
            n40 = Build Array (concatenate)(w115, w116) -> (w113:string[])
            n41 = Build Array (concatenate)(w111, w110) -> (w112:string[])
          }
          n42 = for {
            shift-right: [w106] -> w33
            shift-left: w43 -> [w108]
            tunnel: w34 -> [w107] mode=indexing
            shift-right: [w105] -> w32
            shift-left: w41 -> [w104]
            n43 = Unbundle By Name(w107) -> ("Process Name"=w109:string, "Queue Name"=w103:string)
            n44 = Build Array (concatenate)(w108, w109) -> (w106:string[])
            n45 = Build Array (concatenate)(w104, w103) -> (w105:string[])
          }
          n46 = for {
            shift-right: [w99] -> w21
            shift-left: w33 -> [w101]
            tunnel: w31 -> [w100] mode=indexing
            shift-right: [w98] -> w17
            shift-left: w32 -> [w97]
            n47 = Unbundle By Name(w100) -> ("Process Name"=w102:string, "Queue Name"=w96:string)
            n48 = Build Array (concatenate)(w101, w102) -> (w99:string[])
            n49 = Build Array (concatenate)(w97, w96) -> (w98:string[])
          }
          n50 = for {
            shift-right: [w92] -> w18
            shift-left: w21 -> [w94]
            tunnel: w20 -> [w93] mode=indexing
            shift-right: [w91] -> w16
            shift-left: w17 -> [w90]
            n51 = Unbundle By Name(w93) -> ("Process Name"=w95:string, "Queue Name"=w89:string)
            n52 = Build Array (concatenate)(w94, w95) -> (w92:string[])
            n53 = Build Array (concatenate)(w90, w89) -> (w91:string[])
          }
          n54 = for {
            shift-right: [w85] -> w14
            shift-left: w18 -> [w87]
            tunnel: w19 -> [w86] mode=indexing
            shift-right: [w84] -> w15
            shift-left: w16 -> [w83]
            n55 = Unbundle By Name(w86) -> ("Process Name"=w88:string, "Queue Name"=w82:string)
            n56 = Build Array (concatenate)(w87, w88) -> (w85:string[])
            n57 = Build Array (concatenate)(w83, w82) -> (w84:string[])
          }
          n58 = Build Array (concatenate)("Default", "Start Loop", "End Loop", w15) -> (w35:string[])
          n59 = Build Array (concatenate)("Default", "Start Loop", "End Loop", w14) -> (w29:string[])
          n60 = Index Array(array=w69, index #1=0 ("Index"), index #2=1 ("Index"), index #3=2 ("index"), index #4=3 ("index"), index #5=4 ("index"), index #6=5 ("index")) -> (element #3=w67:refnum<vi>)  [unwired: 5 out]
          n61 = Flatten To XML(anything=w29) -> (xml string=w23:string)
          n62 = To More Specific Class(target class=w68, reference=w67) -> (specific class reference=w66:refnum<vi>, error out=w65:errorcluster)  [unwired: 1 in]
          n63 = Search and Replace String(replace all?=TRUE ("replace all? (F)"), input string=w23, search string="\r\n", replace string="_" ("replace string (\"\")")) -> (result string=w24:string)  [unwired: 4 in, 3 out]
          n64 = property class="Ring"(reference=w66, error in=w65, "Strings []"=w29) -> ()  [unwired: 2 out]
          n65 = Build Array (concatenate)(string[] ["Get Sequence Strings"] ("Line of Events"), w24) -> (w22:string[])
          n66 = call "Generate Temporary Report.vi"("Line of Events"=w22, "Module Name"="Sequencer") -> ()  [unwired: 9 in, 1 out]
        }
        frame #1 {
          # "If the Sequencer is not populated load it empty"
          # "If the Sequencer is already populated, load it"
          n67 = Unbundle By Name(w172) -> ("Main Config.Steps"=w173:T1)
          "Main Config.Steps" <- w173
          n68 = for {
            tunnel: w173 -> [w197] mode=indexing
            tunnel: [w196] -> w181 mode=indexing
            tunnel: w166 -> [w188]
            n69 = Unbundle By Name(w197) -> ("Module"=w190:string, "Control"=w195:u16, "Value"=w194:dbl, "Wait (sec)"=w193:dbl)
            n70 = local read "Step Array"() -> (w192:T78[])
            n71 = Search 1D Array(1D array=w188, element=w190) -> (index of element=w189:i32)  [unwired: 1 in]
            n72 = Index Array(array=w192) -> (element=w191:T78)  [unwired: 1 in]
            n73 = Bundle By Name(cluster=w191, "Module"=w189, "Control"=w195, "Value"=w194, "Wait (sec)"=w193) -> (w196:T78)
            "Strings []" <- w188
          }
          n74 = Empty Array?(array=w181) -> (empty?=w182:bool)
          n75 = flat-sequence {
            tunnel: [w183] -> w170
            tunnel: w170 -> [w184]
            tunnel: [w184] -> w169
            tunnel: [w186] -> w171
            tunnel: w169 -> [w185]
            tunnel: [w185] -> w168
            tunnel: w168 -> [w187]
            frame #0 {
              n76 = local read "Step Array"() -> (w183:T78[])
            }
            frame #1 {
              n77 = invoke on="Step Array" class="Arr" method="Reinit To Default"() -> ()  [unwired: 3 in, 3 out]
            }
            frame #2 {
              n78 = local read "Step Array"() -> (w186:T78[])
            }
            frame #3 {
              n79 = local write "Step Array"(w187) -> ()
            }
          }
          n80 = Select(t=w171, s=w182, f=w181) -> (s? t:f=w167:T78[])
          n81 = Array Size(array=w167) -> (size(s)=w180:i32)
          n82 = Max & Min(x=w180, y=w179) -> (min(x,y)=w175:u32)  [unwired: 1 out]
          n83 = Greater?(x=w175, y=u32 1) -> (0:w177:bool)
          n84 = property on="Step Array" class="Arr"("Number of Rows"=w175, "HorizScroll"=FALSE ("Horizontal Scrollbar Visible"), "VertScroll"=w177, "Index Values"=u32[] [0], "Value"=w167) -> ()  [unwired: 2 in, 2 out]
        }
        frame #2 {
          n85 = invoke class="VI" method="FP.Open"() -> ()  [unwired: 5 in, 5 out]
        }
        frame #3 {
          n86 = while {
            tunnel: w202 -> [w210]
            shift-right: [w205] -> _
            shift-left: _ -> [w204]
            tunnel: [w203] -> w200
            stop <- w208 stop-if-true
            n87 = event shown="[0] \"Step Array\": Value Change" {
              selector: _ -> [_ _ _ _ _ _]
              dyn-events: _ -> [_ _ _ _ _ _]
              timeout: _ -> [_ _ _ _ _ _]
              tunnel: [_ "Start Button" "Cancel Button" "Abort  Button" TRUE ("Save Button") "Save Button"] -> w208
              tunnel: w210 -> [w214 _ _ _ _ _]
              tunnel: [_ _ "Cancel Button" _ _ _] -> w209
              tunnel: [_ "Start Button" _ _ _ _] -> w207
              tunnel: [_ _ _ _ "Pause Button" _] -> w206
              tunnel: [w212 w258 w262 w267 w270 w275] -> w205
              tunnel: w204 -> [_ w258 w262 w267 w270 w275]
              tunnel: [_ _ _ "Abort  Button" _ _] -> w203
              event "Step Array": Value Change {
                n88 = event-data() -> ("NewVal"=w211:T78[])  [unwired: 1 in]
                n89 = for {
                  tunnel: w211 -> [w250] mode=indexing
                  tunnel: [w251] -> w224 mode=indexing
                  tunnel: [w252] -> w223 mode=indexing
                  tunnel: [w249] -> w213 mode=indexing
                  workers-P: _ -> [_]
                  n90 = in-place {
                    in-place-border: [w254] -> w252
                    in-place-border: [w255] -> w251
                    w253 = FALSE ("Add Button")
                    n91 = in-place-cluster #1(w250) -> ("Add Button"=w255:bool, "Remove Button"=w254:bool)
                    n92 = in-place-cluster #1("Add Button"=w253, "Remove Button"=w253) -> (w249:T78)
                  }
                }
                n93 = Or Array Elements(Boolean array=w224) -> (logical OR=w225:bool)
                n94 = Or Array Elements(Boolean array=w223) -> (logical OR=w222:bool)
                n95 = case "Add?" shown="False" w225 {
                  tunnel: w224 -> [_ w248]
                  tunnel: w213 -> [w232 w246]
                  tunnel: [w231 w244] -> w212
                  tunnel: w223 -> [w234 _]
                  tunnel: w222 -> [w233 _]
                  tunnel: [_ w243] -> w215
                  frame False {
                    n96 = case "Remove?" shown="True" w233 {
                      tunnel: w234 -> [_ w240]
                      tunnel: w232 -> [w235 w239]
                      tunnel: [w235 w236] -> w231
                      frame False {
                      }
                      frame True {
                        n97 = Search 1D Array(1D array=w240, element=TRUE) -> (index of element=w237:i32)  [unwired: 1 in]
                        n98 = Delete From Array(array=w239, length=1, index=w237) -> (array with subset deleted=w236:T78[])  [unwired: 1 out]
                      }
                    }
                  }
                  frame True {
                    n99 = Search 1D Array(1D array=w248, element=TRUE) -> (index of element=w245:i32)  [unwired: 1 in]
                    n100 = Increment(x=w245) -> (x+1=w243:i32)
                    n101 = Insert Into Array(array=w246, index=w243, new element=T79 {"Add Button"=FALSE, "Remove Button"=FALSE, "Module"=0, "Control"=9, "Value"=0.0, "Wait (sec)"=0.0, "Step Running"=FALSE} ("Add/Remove Cluster")) -> (w244:T78[])
                  }
                }
                n102 = local write "Step Array"(w212) -> ()
                n103 = Greater Or Equal?(x=w215, y=w214) -> (x >= y?=w216:bool)
                n104 = Array Size(array=w212) -> (size(s)=w221:i32)
                n105 = case shown="True" w216 {
                  tunnel: w215 -> [_ w230]
                  tunnel: w214 -> [_ w229]
                  frame False {
                  }
                  frame True {
                    # "Keep last row in view"
                    n106 = Subtract(x=w230, y=w229) -> (x-y=w228:u32)
                    n107 = Increment(x=w228) -> (x+1=w227:u32)
                    n108 = Build Array(w227) -> (w226:u32[])
                    n109 = property on="Step Array" class="Arr"("Index Values"=w226) -> ()  [unwired: 2 in, 2 out]
                  }
                }
                n110 = Max & Min(x=w221, y=w214) -> (min(x,y)=w218:u32)  [unwired: 1 out]
                n111 = Greater?(x=w218, y=u32 1) -> (0:w217:bool)
                n112 = property on="Step Array" class="Arr"("Number of Rows"=w218, "HorizScroll"=FALSE ("Horizontal Scrollbar Visible"), "VertScroll"=w217) -> ()  [unwired: 2 in, 2 out]
              }
              event "Start Button": Value Change {
                n113 = event-data() -> ()  [unwired: 1 in, 1 out]
                n114 = call "Generate Temporary Report.vi"("Line of Events"=string[] ["Started"], "Module Name"="Sequencer") -> ()  [unwired: 9 in, 1 out]
              }
              event "Cancel Button": Value Change {
                n115 = event-data() -> ()  [unwired: 1 in, 1 out]
                n116 = call "Generate Temporary Report.vi"("Line of Events"=string[] ["Canceled"], "Module Name"="Sequencer") -> ()  [unwired: 9 in, 1 out]
              }
              event "Abort  Button": Value Change {
                n117 = event-data() -> ()  [unwired: 1 in, 1 out]
                n118 = call "Generate Temporary Report.vi"("Line of Events"=string[] ["Aborted"], "Module Name"="Sequencer") -> ()  [unwired: 9 in, 1 out]
              }
              event "Pause Button": Value Change {
                n119 = event-data() -> ()  [unwired: 1 in, 1 out]
                n120 = call "Generate Temporary Report.vi"("Line of Events"=string[] ["Paused"], "Module Name"="Sequencer") -> ()  [unwired: 9 in, 1 out]
              }
              event "Save Button": Value Change {
                n121 = event-data() -> ()  [unwired: 1 in, 1 out]
                n122 = call "Generate Temporary Report.vi"("Line of Events"=string[] ["Saved"], "Module Name"="Sequencer") -> ()  [unwired: 9 in, 1 out]
              }
            }
            "cancelled" <- w209
            "Start" <- w207
            "Pause" <- w206
            "Abort" <- w203
          }
        }
        frame #4 {
          n123 = local read "cancelled"() -> (w283:bool)
          n124 = case shown="False" w283 {
            tunnel: w281 -> [w297 w310]
            tunnel: [w296 w310] -> w282
            tunnel: w281 -> [w295 _]
            tunnel: w279 -> [w294 _]
            tunnel: w278 -> [w293 _]
            frame False {
              # "Send out the Sequence"
              n125 = local read "Step Array"() -> (w298:T78[])
              n126 = for {
                tunnel: w298 -> [w309] mode=indexing
                tunnel: [w305] -> w284 mode=indexing
                tunnel: w295 -> [w300]
                tunnel: w293 -> [w299]
                n127 = Unbundle By Name(w300) -> ("Main Config.Steps"=w304:T1)
                n128 = Unbundle By Name(w309) -> ("Module"=w302:u16, "Control"=w308:u16, "Value"=w307:dbl, "Wait (sec)"=w306:dbl)
                n129 = property on="Module" class="Ring (strict)" props=["Strings []"]() -> ()  [unwired: 2 in, 3 out]
                n130 = Index Array(array=w304) -> (element=w303:T2)  [unwired: 1 in]
                n131 = Index Array(array=w299, index=w302) -> (element=w301:string)
                n132 = Bundle By Name(cluster=w303, "Module"=w301, "Control"=w308, "Value"=w307, "Wait (sec)"=w306) -> (w305:T2)
              }
              "Steps out" <- w284
              n133 = Bundle By Name(cluster=w297, "Main Config.Abort"=w294, "Main Config.Steps"=w284) -> (w296:T3)
              n134 = Flatten To XML(anything=w284) -> (xml string=w291:string)
              n135 = Search and Replace String(replace all?=TRUE ("replace all? (F)"), input string=w291, search string="\r\n", replace string="_" ("replace string (\"\")")) -> (result string=w290:string)  [unwired: 4 in, 3 out]
              n136 = Build Array (concatenate)(string[] ["Steps Accepted"] ("Line of Events"), w290) -> (w292:string[])
              n137 = call "Generate Temporary Report.vi"("Line of Events"=w292, "Module Name"="Sequencer") -> ()  [unwired: 9 in, 1 out]
            }
            frame True {
            }
          }
          n138 = invoke class="VI" method="FP.Close"() -> ()  [unwired: 3 in, 3 out]
          n139 = call-poly "Enqueue Message.vi"("Message"="Exit", "Message Queue"=w277) -> ()  [unwired: 8 in, 2 out]
        }
      }
    }
    frame Error {
    }
  }
  "error out" <- w7
  "State Cluster Out" <- w5
  n140 = while {
    tunnel: "Sequence UI" -> [w317]
    stop <- w316 stop-if-true
    n141 = call "Dequeue Message.vi"("Message Queue"=w317) -> ("Message Data"=w315:variant, "Message"=w318:string)  [unwired: 7 in, 2 out]
    n142 = Variant To Data(type=0, Variant=w315) -> (data=w313:i32)  [unwired: 1 in, 1 out]
    n143 = case shown="\"Update Step\"" w318 {
      tunnel: [FALSE FALSE TRUE] -> w316
      tunnel: w313 -> [_ w322 _]
      frame Default {
        n144 = Wait (ms)(milliseconds to wait=u32 50) -> ()  [unwired: 1 out]
      }
      frame "Update Step" {
        n145 = local read "Step Array"() -> (w323:T78[])
        n146 = for {
          tunnel: w323 -> [w327] mode=indexing
          tunnel: w322 -> [w328]
          tunnel: [w326] -> w321 mode=indexing
          i -> [w329]
          n147 = Equal?(x=w329, y=w328) -> (x = y?=w325:bool)
          n148 = Bundle By Name(cluster=w327, "Step Running"=w325) -> (w326:T78)
        }
        n149 = local write "Step Array"(w321) -> ()
      }
      frame "Exit" {
      }
    }
  }
